vi "lib Space Delimited String to Array.vi"(4 "String":string) -> (1 "Array":string[](array[string]))   [LabVIEW 2015]
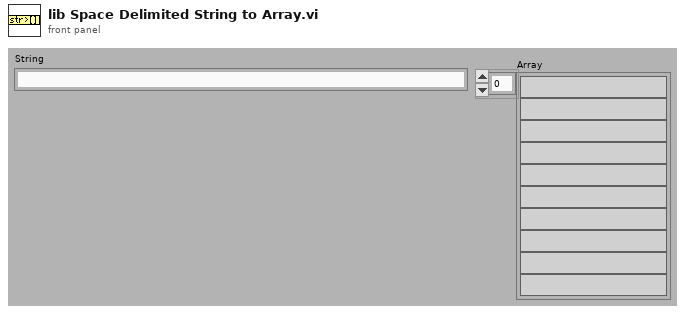
[diagram p1: front panel]
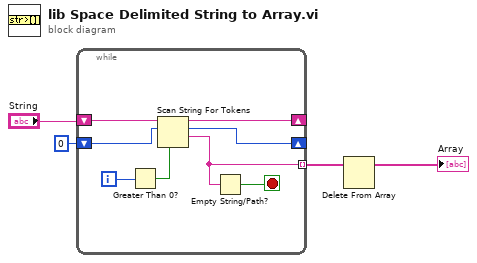
[diagram p0: block diagram]
diagram:
  n1 = while {
    shift-right: [w8] -> _
    shift-left: "String" -> [w12]
    shift-right: [w9] -> _
    shift-left: 0 ("offset past token") -> [w10]
    tunnel: [w5] -> w3 mode=indexing
    i -> [w11]
    stop <- w7 stop-if-true
    n2 = Greater Than 0?(x=w11) -> (x > 0?=w6:bool)
    n3 = Scan String For Tokens(4:w6, 8:w10, 9:w12) -> (1:w5:string, 2:w9:i32, 3:w8:string)  [unwired: 3 in, 1 out]
    n4 = Empty String/Path?(string/path=w5) -> (empty?=w7:bool)
  }
  n5 = Delete From Array(array=w3) -> (array with subset deleted=→"Array":string[])  [unwired: 2 in, 1 out]
